vi "Read Jitter Measurement (Clock TIE).vi"(6 "Slope Clock TIE (0: Rising)":u16(ring) items=["Rising", "Falling", "Both"], 8 "error in (no error)":errorcluster, 9 "Units Clock TIE (0: Seconds)":u16(ring) items=["Seconds", "Unit Interval"], 10 "Source Clock TIE (0: Channel 1)":u16(ring) items=["Channel 1", "Channel 2", "Channel 3", "Channel 4", "Math 1", "Math 2", "Math 3", "Math 4", "Reference Waveform 1", "Reference Waveform 2", "Reference Waveform 3", "Reference Waveform 4"], 11 "VISA resource name":refnum<visa-resource-name>) -> (0 "error out":errorcluster, 2 "Clock TIE":dbl, 3 "VISA resource name out":refnum<visa-resource-name>)   [LabVIEW 2016, in "Agilent 2000 3000 X-Series.lvlib"]
doc: "Measures and returns the Clock TIE jitter value.\n\n<b>Note:</b>\nThis VI is specific to the 6000-X Series oscilloscopes. These features are not available on other models."
uses:
  Agilent 2000 3000 X-Series.lvlib
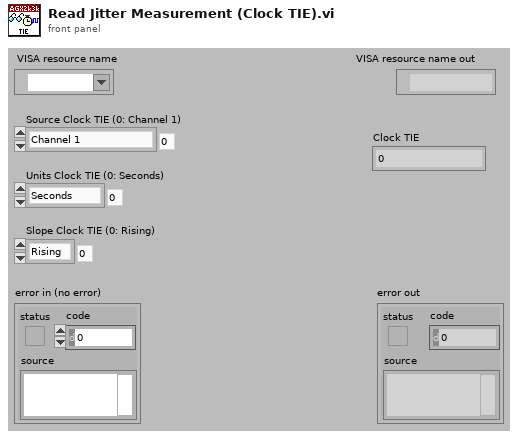
[diagram p1: front panel]
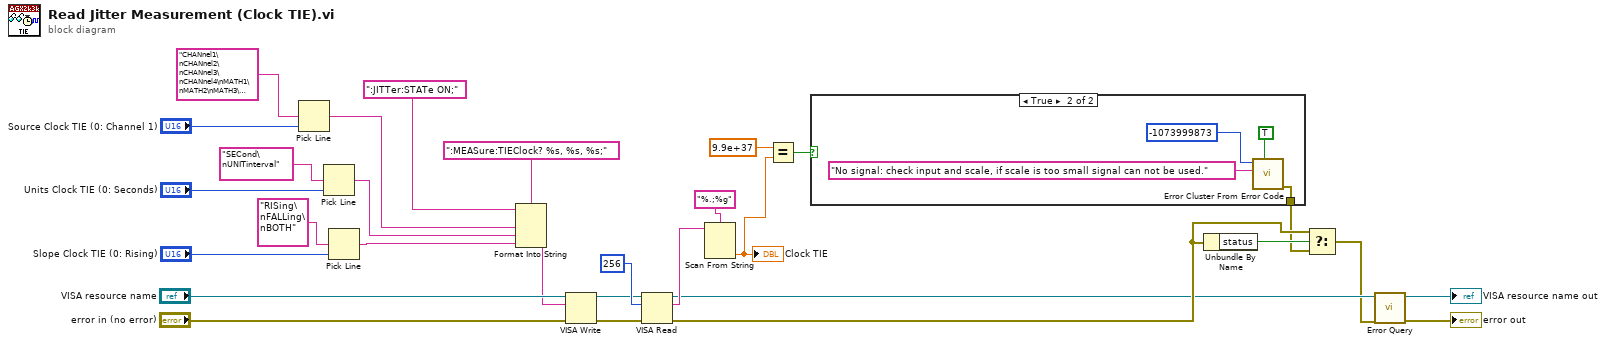
[diagram p0: block diagram]
diagram:
  n1 = Pick Line(multi-line string="CHANnel1\nCHANnel2\nCHANnel3\nCHANnel4\nMATH1\nMATH2\nMATH3\nMATH4\nWMEMory1\nWMEMory2\nWMEMory3\nWMEMory4", line index="Source Clock TIE (0: Channel 1)") -> (output string=w26:string)  [unwired: 1 in]
  n2 = Pick Line(multi-line string="SECond\nUNITinterval", line index="Units Clock TIE (0: Seconds)") -> (output string=w23:string)  [unwired: 1 in]
  n3 = Pick Line(multi-line string="RISing\nFALLing\nBOTH", line index="Slope Clock TIE (0: Rising)") -> (output string=w20:string)  [unwired: 1 in]
  n4 = Format Into String(format string=":MEASure:TIEClock? %s, %s, %s;", initial string=":JITTer:STATe ON;", w26, w23, w20) -> (resulting string=w14:string)  [unwired: 1 in, 1 out]
  n5 = VISA Write(VISA resource name="VISA resource name", write buffer=w14, error in (no error)="error in (no error)") -> (VISA resource name out=w4:refnum<visa-resource-name>, error out=w3:errorcluster)  [unwired: 1 out]
  n6 = VISA Read(VISA resource name=w4, byte count=u32 256, error in (no error)=w3) -> (VISA resource name out=w2:refnum<visa-resource-name>, read buffer=w13:string, error out=w7:errorcluster)  [unwired: 1 out]
  n7 = Scan From String(format string="%.;%g", input string=w13) -> (output 1=w9:dbl)  [unwired: 3 in, 3 out]
  "Clock TIE" <- w9
  n8 = Equal?(x=9.9e+37, y=w9) -> (x = y?=w11:bool)
  n9 = case shown="True" w11 {
    tunnel: [_ w30] -> w6
    frame False {
    }
    frame True {
      n10 = call <vilib>:"Error Cluster From Error Code.vi"("show call chain? (False)"=TRUE, "error message (\"\")"="No signal: check input and scale, if scale is too small signal can not be used." ("error message (\"\")"), "error code (0)"=-1073999873) -> ("error out"=w30:errorcluster)  [unwired: 6 in]
    }
  }
  n11 = Unbundle By Name(w7) -> ("status"=w8:bool)
  n12 = Select(t=w7, s=w8, f=w6) -> (s? t:f=w1:errorcluster)
  n13 = call "Error Query.vi"("error in (no error)"=w1, "VISA resource name"=w2) -> ("error out"=→"error out":errorcluster, "VISA resource name out"=→"VISA resource name out":refnum<visa-resource-name>)  [unwired: 6 in, 2 out]
